vi "TCP 서버.vi"() -> ()   [LabVIEW 2014]
uses:
  <vilib>/Analysis/NI_AALBase.lvlib
panel:
  out "숫자형":i32
  out "에러 출력":errorcluster
  out "웨이브폼 그래프":dbl[](graph)
  in  "정지":bool
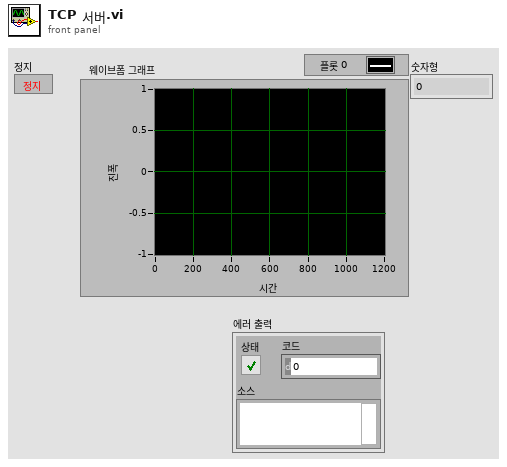
[diagram p1: front panel]
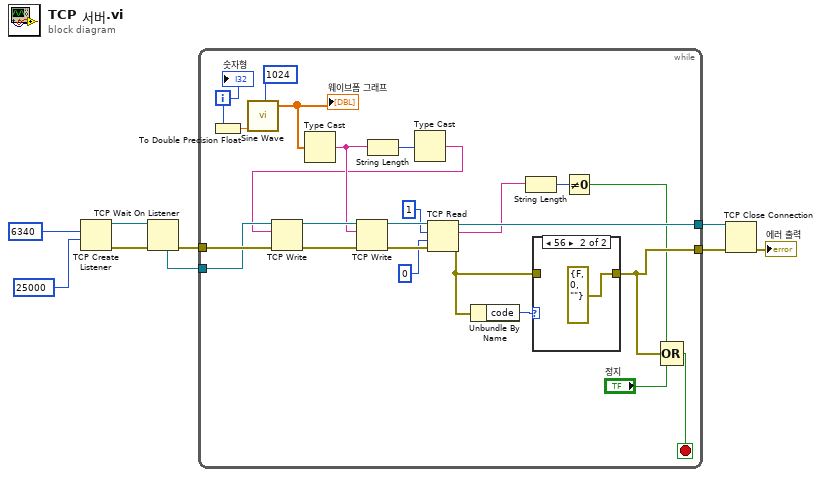
[diagram p0: block diagram]
diagram:
  n1 = TCP Create Listener(9:25000 ("타임아웃 ms (25000)"), 10:u16 6340 ("포트")) -> (0:w8:errorcluster, 3:w9:refnum<k5>)  [unwired: 3 in, 1 out]
  n2 = TCP Wait On Listener(8:w8, 11:w9) -> (0:w5:errorcluster, 4:w4:refnum<k5>)  [unwired: 2 in, 3 out]
  n3 = while {
    tunnel: w5 -> [w33]
    tunnel: w4 -> [w32]
    tunnel: [w25] -> w3
    tunnel: [w21] -> w2
    i -> [w16]
    stop <- w22 stop-if-true
    n4 = To Double Precision Float(number=w16) -> (double precision float=w15:dbl)
    n5 = call <vilib>:"Sine Wave.vi"("samples"=1024, "phase in"=w15) -> ("sine wave"=w14:dbl[])  [unwired: 3 in, 2 out]
    "웨이브폼 그래프" <- w14
    n6 = Type Cast(x=w14) -> (*(type *) &x=w13:string)  [unwired: 1 in]
    n7 = String Length(string=w13) -> (length=w12:i32)
    n8 = Type Cast(x=w12) -> (*(type *) &x=w11:string)  [unwired: 1 in]
    n9 = TCP Write(connection ID=w32, data in=w11, error in (no error)=w33) -> (connection ID out=w31:refnum<k5>, error out=w30:errorcluster)  [unwired: 1 in, 1 out]
    n10 = TCP Write(connection ID=w31, data in=w13, error in (no error)=w30) -> (connection ID out=w29:refnum<k5>, error out=w28:errorcluster)  [unwired: 1 in, 1 out]
    n11 = TCP Read(connection ID=w29, bytes to read=1 ("읽을 바이트"), error in (no error)=w28, 9:0 ("타임아웃 ms (25000)")) -> (connection ID out=w25:refnum<k5>, data out=w19:string, error out=w23:errorcluster)  [unwired: 1 in]
    n12 = Unbundle By Name(w23) -> ("code"=w24:i32)
    n13 = String Length(string=w19) -> (length=w18:i32)
    n14 = case shown="56" w24 {
      tunnel: w23 -> [w34 _]
      tunnel: [w34 errorcluster {"status"=FALSE, "code"=0, "source"=""} ("에러 상수")] -> w21
      frame 0, Default {
      }
      frame 56 {
      }
    }
    n15 = Not Equal To 0?(x=w18) -> (x != 0?=w17:bool)
    n16 = Compound Arithmetic op=OR(w17, w21, "정지") -> (w22:bool)
    "숫자형" <- w16
  }
  n17 = TCP Close Connection(connection ID=w3, error in (no error)=w2) -> (error out=→"에러 출력":errorcluster)  [unwired: 1 in, 1 out]
